vi "2022_day08.vi"() -> ()   [LabVIEW 2021]
uses:
  <userlib>/_OpenG.lib/array/array.llb/Reverse 2D Array (I32)__ogtk.vi
  <userlib>/_OpenG.lib/array/array.llb/Reverse 2D Array (Boolean)__ogtk.vi
panel:
  out "Task 2":i32
  out "Task 1":i16
  in  "Switch":bool caption="Ex. Data  vs.  User Data"
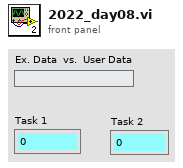
[diagram p1: front panel]
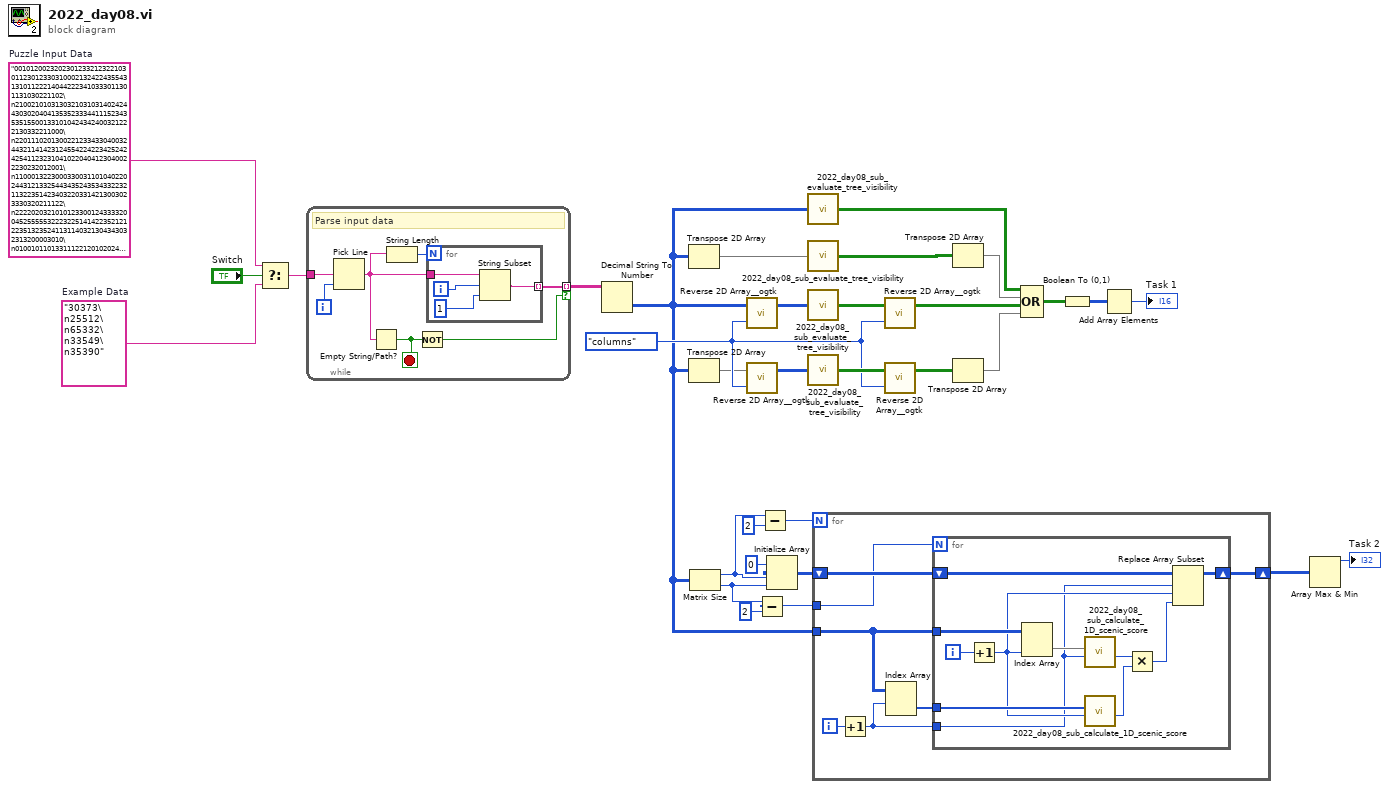
[diagram p0: block diagram]
diagram:
  w18 = enum16{"rows", "columns"}."columns" ("by rows or columns (rows)")
  w31 = "001012002320230123321232210301123012330310002132422435543131011222140442223410333011301131030221102\n210021010313032103103140242443030204041353523334411152343535155001331010424342400321222130332211000\n220111020130022123343304003244321141423124554224223425242425411232310410220404123040022230232012001\n110001322300033003110104022024431213325443435243534332232113223514234032203314213003023330320211122\n222202032101012330012433332004525555532223225141422352121223513235241131140321304343032313200003010\n010010110133111221201020242055234235524542112413124323131144113543431153434301004404433332201031101\n..."  # Puzzle Input Data
  w30 = "30373\n25512\n65332\n33549\n35390"  # Example Data
  n1 = Select(t=w31, s="Switch", f=w30) -> (s? t:f=w29:string)
  n2 = while {
    tunnel: w29 -> [w39]
    tunnel: [w36] -> w28 mode=indexing if=w33
    i -> [w35]
    stop <- w34 stop-if-true
    # "Parse input data"
    n3 = Pick Line(multi-line string=w39, line index=w35) -> (output string=w37:string)  [unwired: 1 in]
    n4 = Empty String/Path?(string/path=w37) -> (empty?=w34:bool)
    n5 = String Length(string=w37) -> (length=w38:i32)
    n6 = Not(x=w34) -> (.not. x?=w33:bool)
    n7 = for {
      N: w38 -> [_]
      tunnel: w37 -> [w43]
      tunnel: [w41] -> w36 mode=indexing
      i -> [w40]
      n8 = String Subset(string=w43, offset (0)=w40, length (rest)=1 ("length (rest)")) -> (substring=w41:string)
    }
  }
  n9 = Decimal String To Number(string=w28) -> (number=w10:i32[][])  [unwired: 2 in, 1 out]
  n10 = Transpose 2D Array(2D array=w10) -> (transposed array=w27:i32[][])
  n11 = Transpose 2D Array(2D array=w10) -> (transposed array=w17:i32[][])
  n12 = Matrix Size(0:w10) -> (1:w8:i32, 2:w5:i32)
  n13 = call-poly <userlib>:"Reverse 2D Array__ogtk.vi"("by rows or columns (rows)"=w18, "Array"=w10) -> ("Reversed Array"=w23:i32[][])  [unwired: 1 in]
  n14 = call-poly <userlib>:"Reverse 2D Array__ogtk.vi"("by rows or columns (rows)"=w18, "Array"=w17) -> ("Reversed Array"=w19:i32[][])  [unwired: 1 in]
  n15 = Subtract(x=w5, y=2 ("x")) -> (x-y=w4:i32)
  n16 = Subtract(x=w8, y=2 ("x")) -> (x-y=w9:i32)
  n17 = Initialize Array(0 ("length (rest)"), w8, w5) -> (w3:i32[][])
  n18 = call "2022_day08_sub_evaluate_tree_visibility.vi"("Tree Sizes Map"=w10) -> ("Visible Trees Map"=w25:bool[][])
  n19 = call "2022_day08_sub_evaluate_tree_visibility.vi"("Tree Sizes Map"=w27) -> ("Visible Trees Map"=w26:bool[][])
  n20 = call "2022_day08_sub_evaluate_tree_visibility.vi"("Tree Sizes Map"=w23) -> ("Visible Trees Map"=w22:bool[][])
  n21 = call "2022_day08_sub_evaluate_tree_visibility.vi"("Tree Sizes Map"=w19) -> ("Visible Trees Map"=w20:bool[][])
  n22 = for {
    N: w9 -> [_]
    tunnel: w10 -> [w46]
    tunnel: w4 -> [w48]
    shift-right: [w49] -> w2
    shift-left: w3 -> [w50]
    i -> [w47]
    n23 = Increment(x=w47) -> (x+1=w45:i32)
    n24 = Index Array(array=w46, index (row)=w45) -> (element=w44:i32[])  [unwired: 1 in]
    n25 = for {
      N: w48 -> [_]
      tunnel: w46 -> [w61]
      tunnel: w45 -> [w51]
      shift-right: [w58] -> w49
      shift-left: w50 -> [w60]
      tunnel: w44 -> [w56]
      i -> [w59]
      n26 = Increment(x=w59) -> (x+1=w52:i32)
      n27 = Index Array(array=w61, index (col)=w52) -> (element=w57:i32[])  [unwired: 1 in]
      n28 = call "2022_day08_sub_calculate_1D_scenic_score.vi"("Element Idx"=w51, "Array In"=w57) -> ("Result"=w55:i32)  [unwired: 9 in]
      n29 = call "2022_day08_sub_calculate_1D_scenic_score.vi"("Element Idx"=w52, "Array In"=w56) -> ("Result"=w54:i32)  [unwired: 9 in]
      n30 = Multiply(x=w55, y=w54) -> (x*y=w53:i32)
      n31 = Replace Array Subset(array=w60, new element=w53, index (row)=w51, index (col)=w52) -> (w58:i32[][])
    }
  }
  n32 = call-poly <userlib>:"Reverse 2D Array__ogtk.vi"("by rows or columns (rows)"=w18, "Array"=w22) -> ("Reversed Array"=w21:bool[][])  [unwired: 1 in]
  n33 = call-poly <userlib>:"Reverse 2D Array__ogtk.vi"("by rows or columns (rows)"=w18, "Array"=w20) -> ("Reversed Array"=w16:bool[][])  [unwired: 1 in]
  n34 = Transpose 2D Array(2D array=w26) -> (transposed array=w24:bool[][])
  n35 = Transpose 2D Array(2D array=w16) -> (transposed array=w15:bool[][])
  n36 = Compound Arithmetic op=OR(w25, w24, w21, w15) -> (w14:bool[][])
  n37 = Boolean To (0,1)(Boolean=w14) -> (0, 1=w13:i16[][])
  n38 = Add Array Elements(numeric array=w13) -> (sum=→"Task 1":i16)
  n39 = Array Max & Min(array=w2) -> (max value=→"Task 2":i32)  [unwired: 3 out]
